vi "Initialise.vi"(8 "error in (no error)":errorcluster, 10 "Message in":refnum<class "InitialiseMessage.lvclass">, 11 "Autofocus in":refnum<class "Autofocus.lvclass">) -> (0 "error out":errorcluster, 3 "Autofocus out":refnum<class "Autofocus.lvclass">)   [LabVIEW 2012, in "Autofocus.lvclass"]
doc: "This method is called when an initialise message is received. It mainly initialises the RabbitMQ connectivity. \n\nOverride this method when your component needs special initialisation (e.g. of software or hardware resources). In that case, don't forget to call the parent for proper implementation. If your component owns subcomponents, they count as resources, so you have to initialise them by calling their own initialise functions"
uses:
  Autofocus.lvclass
  <vilib>/Distrio/Murmex/InitialiseMessage/InitialiseMessage.lvclass
  <vilib>/Distrio/Murmex/Murmex/Murmex.lvclass
  Hill Climbing.ctl
  Golden Section.ctl
  checkpoint.ctl
  stack.ctl
  settings cluster.ctl
  Sharpness Measure.ctl
  ROI size.ctl
  Search algorithm.ctl
  image acquisition mode.ctl
  Tomo.ctl
  Autofocus.lvclass/Autofocus.ctl
panel:
  # "This method is called when the INTIALISE\ntrigger is sent. \n\nOverride this method when your component needs to\nrespond to this trigger. \n\nCall parent for proper implementation"
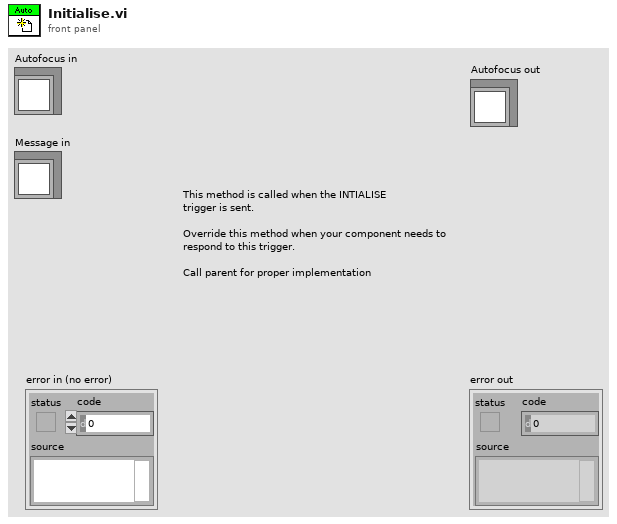
[diagram p1: front panel]
types:
  T1 = typedef "Autofocus.lvclass/Tomo.ctl" = cluster{"stack counter":dbl, "slope array":dbl[], "intercept array":dbl[], "z_start array":dbl[], "z_stop array":dbl[], "Interpolation data":dbl[][][], "progress":dbl}
  T2 = typedef "Autofocus.lvclass/settings cluster.ctl" = cluster{"Sharpness measure":T3, "ROI size":T4, "Search Algorithm":T5, "Region sampling":bool, "HC step size":dbl[unit], "current_position_focus":dbl[unit], "threshold":dbl, "brightest percentage":dbl, "numer_of_frames":u16, "number_of_checkpoints":u16, "current_stack_x":dbl[unit], "current_stack_y":dbl[unit], "curent_stack_z1":dbl[unit], "current_stack_z2":dbl[unit], "number_of_stacks":u16, "focus_start":dbl[unit], "focus_stop":dbl[unit], "frames_focus_stack":u16, "Image acquisition mode":T6}
  T3 = typedef "Autofocus.lvclass/Sharpness Measure.ctl" = enum16{"Vol4", "Gradient Square"}
  T4 = typedef "Autofocus.lvclass/ROI size.ctl" = u16
  T5 = typedef "Autofocus.lvclass/Search algorithm.ctl" = enum16{"Hill Climbing", "HC+GS"}
  T6 = typedef "Autofocus.lvclass/image acquisition mode.ctl" = enum16{"Focus Stack", "Single Frame"}
  T7 = typedef "Autofocus.lvclass/stack.ctl" = cluster{"checkpoint counter":i32, "starting time":dbl, "above threshold?":bool, "intercept":dbl, "slope":dbl, "z_start":dbl[unit], "z_stop":dbl[unit], "focus positions":dbl[], "stage positions":dbl[], "progress":dbl, "do autofocusing?":bool}
  T8 = typedef "Autofocus.lvclass/checkpoint.ctl" = cluster{"max image sharpness ":dbl, "iteration number":i32, "starting time":dbl, "Image sharpness array":dbl[], "current image sharpness":dbl, "Image sharpness n-1":dbl, "defocus positions":dbl[]}
  T9 = cluster{"f(a)":dbl, "f(b)":dbl, "f(c)":dbl, "f(d)":dbl}
  T10 = cluster{"lower limit a":dbl[unit], "upper limit b":dbl[unit], "point c":dbl[unit], "point d":dbl[unit]}
  T11 = typedef "Autofocus.lvclass/Golden Section.ctl" = cluster{"current range":cluster{"lower limit a":dbl[unit], "upper limit b":dbl[unit], "point c":dbl[unit], "point d":dbl[unit]}, "Sharpness points":cluster{"f(a)":dbl, "f(b)":dbl, "f(c)":dbl, "f(d)":dbl}, "found focus (GS)?":bool}
  T12 = typedef "Autofocus.lvclass/Hill Climbing.ctl" = cluster{"keep direction?":bool, "met downhill?":bool, "first iteration of round?":bool, "HC done?":bool, "found focus (HC)?":bool, "limit switch":bool}
  T13 = typedef "Autofocus.lvclass/number of subregions.ctl" = i32
  T14 = typedef "Image Type" = u32
  T15 = typedef "IMAQ Image.ctl" = refnum<image>
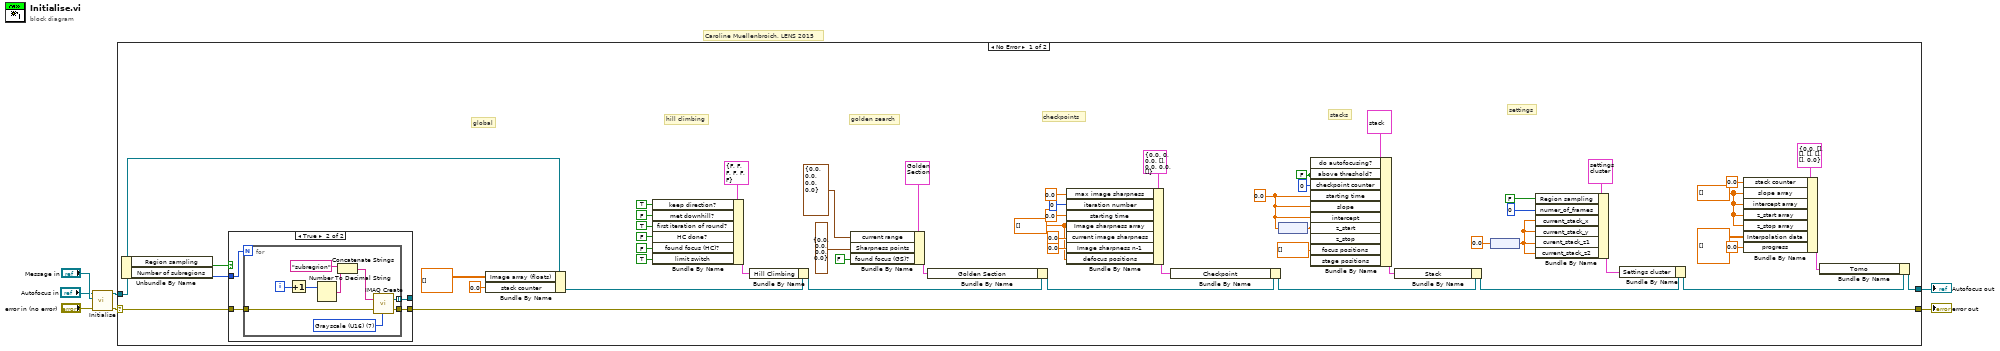
[diagram p0: block diagram]
diagram:
  # "Caroline Muellenbroich, LENS 2015"
  n1 = call-parent "Initialise.vi"("error in (no error)"="error in (no error)", "Message in"="Message in", "Murmex in"="Autofocus in") -> ("error out"=w4:errorcluster, "Murmex out"=w2:refnum<class "Autofocus.lvclass">)  [unwired: 7 in]
  n2 = case shown="No Error" w4 {
    selector: w4 -> [w61 w76]
    tunnel: [w60 w76] -> w3
    tunnel: w2 -> [w59 w77]
    tunnel: [w15 w77] -> w1
    frame No Error {
      w11 = dbl[] [] ("slope array")
      w27 = dbl[] [] ("focus positions")
      w17 = FALSE ("above threshold?")
      w21 = 0.0 ("starting time")
      w28 = dbl[] [] ("Image sharpness array")
      # "settings"
      # "stacks"
      # "checkpoints"
      # "golden search"
      # "hill climbing"
      # "global"
      n3 = Unbundle By Name(w59) -> ("Region sampling"=w58:bool, "Number of subregions"=w57:T13)
      n4 = case shown="True" w58 {
        tunnel: w61 -> [w62 w66]
        tunnel: [w62 w65] -> w60
        tunnel: [_ w64] -> _
        tunnel: w57 -> [_ w63]
        frame False {
        }
        frame True {
          n5 = for {
            N: w63 -> [_]
            tunnel: w66 -> [w70]
            tunnel: [w69] -> w65
            tunnel: [w67] -> w64 mode=indexing
            i -> [w75]
            w68 = T14 7 items=["Grayscale (U8)", "Grayscale (I16)", "Grayscale (SGL)", "Complex (CSG)", "RGB (U32)", "HSL (U32)", "RGB (U64)", "Grayscale (U16)"] ("Image Type")
            n6 = Increment(x=w75) -> (x+1=w73:i32)
            n7 = Number To Decimal String(number=w73) -> (decimal integer string=w72:string)  [unwired: 1 in]
            n8 = Concatenate Strings("subregrion" ("string"), w72) -> (w74:string)
            n9 = call "IMAQ Create"("Image Name"=w74, "Image Type"=w68, "error in (no error)"=w70) -> ("New Image"=w67:T15, "error out"=w69:errorcluster)  [unwired: 2 in]
          }
        }
      }
      n10 = Bundle By Name(cluster=w59, "Image array (floats)"=dbl[][] [] ("Runtime cluster.Image array (floats)"), "stack counter"=0.0 ("Runtime cluster.Tomo.stack counter")) -> (w48:refnum<class "Autofocus.lvclass">)
      n11 = Bundle By Name(cluster=T12 {"keep direction?"=FALSE, "met downhill?"=FALSE, "first iteration of round?"=FALSE, "HC done?"=FALSE, "found focus (HC)?"=FALSE, "limit switch"=FALSE} ("Runtime cluster.Hill Climbing"), "keep direction?"=TRUE, "met downhill?"=FALSE, "first iteration of round?"=TRUE, "HC done?"=FALSE, "found focus (HC)?"=FALSE, "limit switch"=TRUE) -> (w46:T12)
      n12 = Bundle By Name(cluster=w48, "Hill Climbing"=w46) -> (w47:refnum<class "Autofocus.lvclass">)
      n13 = Bundle By Name(cluster=T11 {"current range"={"lower limit a"=0.0, "upper limit b"=0.0, "point c"=0.0, "point d"=0.0}, "Sharpness points"={"f(a)"=0.0, "f(b)"=0.0, "f(c)"=0.0, "f(d)"=0.0}, "found focus (GS)?"=FALSE} ("Runtime cluster.Golden Section"), "current range"=T10 {"lower limit a"=0.0, "upper limit b"=0.0, "point c"=0.0, "point d"=0.0}, "Sharpness points"=T9 {"f(a)"=0.0, "f(b)"=0.0, "f(c)"=0.0, "f(d)"=0.0}, "found focus (GS)?"=FALSE) -> (w44:T11)
      n14 = Bundle By Name(cluster=w47, "Golden Section"=w44) -> (w40:refnum<class "Autofocus.lvclass">)
      n15 = Bundle By Name(cluster=T8 {"max image sharpness "=0.0, "iteration number"=0, "starting time"=0.0, "Image sharpness array"=[], "current image sharpness"=0.0, "Image sharpness n-1"=0.0, "defocus positions"=[]} ("Runtime cluster.Checkpoint"), "max image sharpness"=0.0, "iteration number"=0, "starting time"=0.0, "Image sharpness array"=w28, "current image sharpness"=0.0, "Image sharpness n-1"=0.0, "defocus positions"=w28) -> (w36:T8)
      n16 = Bundle By Name(cluster=w40, "Checkpoint"=w36) -> (w39:refnum<class "Autofocus.lvclass">)
      n17 = node(w21) -> (w20:dbl[unit])
      n18 = Bundle By Name(cluster=T7 {"checkpoint counter"=0, "starting time"=0.0, "above threshold?"=FALSE, "intercept"=0.0, "slope"=0.0, "z_start"=0.0, "z_stop"=0.0, "focus positions"=[], "stage positions"=[], "progress"=0.0, "do autofocusing?"=FALSE} ("Runtime cluster.Stack"), "do autofocusing?"=w17, "above threshold?"=w17, "checkpoint counter"=0 ("iteration number"), "starting time"=w21, "slope"=w21, "intercept"=w21, "z_start"=w20, "z_stop"=w20, "focus positions"=w27, "stage positions"=w27) -> (w35:T7)
      n19 = Bundle By Name(cluster=w39, "Stack"=w35) -> (w26:refnum<class "Autofocus.lvclass">)
      n20 = node(0.0 ("current_stack_x")) -> (w19:dbl[unit])
      n21 = Bundle By Name(cluster=T2 {"Sharpness measure"=enum."Vol4", "ROI size"=0, "Search Algorithm"=enum."Hill Climbing", "Region sampling"=FALSE, "HC step size"=0.0, "current_position_focus"=0.0, "threshold"=0.0, "brightest percentage"=0.0, "numer_of_frames"=0, "number_of_checkpoints"=0, "current_stack_x"=0.0, "current_stack_y"=0.0, "curent_stack_z1"=0.0, "current_stack_z2"=0.0, "number_of_stacks"=0, "focus_start"=0.0, "focus_stop"=0.0, "frames_focus_stack"=0, "Image acquisition mode"=enum."Focus Stack"} ("Settings cluster"), "Region sampling"=FALSE, "numer_of_frames"=u16 0, "current_stack_x"=w19, "current_stack_y"=w19, "curent_stack_z1"=w19, "current_stack_z2"=w19) -> (w24:T2)
      n22 = Bundle By Name(cluster=w26, "Settings cluster"=w24) -> (w16:refnum<class "Autofocus.lvclass">)
      n23 = Bundle By Name(cluster=T1 {"stack counter"=0.0, "slope array"=[], "intercept array"=[], "z_start array"=[], "z_stop array"=[], "Interpolation data"=[], "progress"=0.0} ("Tomo"), "stack counter"=0.0, "slope array"=w11, "intercept array"=w11, "z_start array"=w11, "z_stop array"=w11, "Interpolation data"=dbl[][][] [], "progress"=0.0) -> (w14:T1)
      n24 = Bundle By Name(cluster=w16, "Tomo"=w14) -> (w15:refnum<class "Autofocus.lvclass">)
    }
    frame Error {
    }
  }
  "error out" <- w3
  "Autofocus out" <- w1
